vi "Test Registration.vi"() -> ()   [LabVIEW 2020, in "Scratchpad.lvlib"]
uses:
  Scratchpad.lvlib
  Dummy DB/Dummy DB.lvclass
  C:/dev/lv20CE/lv-conditum/Conditum/Database Platform/Database Platform.lvclass
  Conditum-Example/User/User.lvclass
  C:/dev/lv20CE/lv-conditum/Conditum/Entity/Entity.lvclass
  Conditum/Entity Manager/Entity Manager.lvclass
panel:
  out "error out":errorcluster
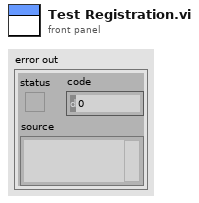
[diagram p1: front panel]
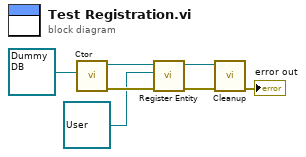
[diagram p0: block diagram]
diagram:
  n1 = call "Ctor.vi"("Database"=refnum<class "Dummy DB.lvclass"> refnum ("Scratchpad.lvlib:Dummy DB.lvclass")) -> ("error out"=w5:errorcluster, "Entity Manager out"=w6:refnum<class "Entity Manager.lvclass">)  [unwired: 9 in]
  n2 = call "Register Entity.vi"("error in (no error)"=w5, "Entity"=refnum<class "User.lvclass"> refnum ("Conditum-Example.lvlib:User.lvclass"), "Entity Manager in"=w6) -> ("error out"=w2:errorcluster, "Entity Manager out"=w3:refnum<class "Entity Manager.lvclass">)  [unwired: 7 in]
  n3 = call "Cleanup.vi"("error in (no error)"=w2, "Entity Manager in"=w3) -> ("error out"=→"error out":errorcluster)  [unwired: 9 in]
